vi "Strategy 5_Autotuning PID Offline.vi"() -> ()   [LabVIEW 2018]
doc: "This example demonstrates how to use the PID Design function to obtain PID parameters based on measured process."
uses:
  <vilib>/DAQmx/write.llb/DAQmx Write (Digital 1D Bool 1Chan 1Samp).vi
  <vilib>/addons/control/pid/autopid.llb/PID Autotuning Design (Ziegler-Nichols).vi
  <vilib>/addons/control/pid/autopid.llb/PID Autotuning Design (Cohen-Coon).vi
  <vilib>/addons/control/pid/autopid.llb/PID Autotuning Design (Chien-Hrones-Reswick).vi
  <vilib>/addons/control/pid/autopid.llb/PID Autotuning Design (Internal Model Control).vi
  <vilib>/DAQmx/create/channels.llb/DAQmx Create Channel (DO-Digital Output).vi
  <vilib>/addons/control/pid/pid.llb/PID Advanced (DBL).vi
  <vilib>/DAQmx/miscellaneous.llb/DAQmx Fill In Error Info.vi
  <vilib>/addons/control/pid/NI_PID_autopid.lvlib
  <vilib>/addons/control/pid/NI_PID_pid.lvlib
  <vilib>/ptbypt/NI_PtbyPt.lvlib
panel:
  out "PWM Output":bool
  out "Waveform Chart 2":dbl[][](graph)
  in  "MV:":dbl(slide)=20.39115328927357 scale=-100.0..100.0
  in  "Set\nPoint":dbl(slide) scale=0.0..30.0
  out "Waveform Chart":dbl[][](graph)
  in  "sample length":i32=100
  in  "Excitation":dbl=0.5 format="%.2f"
  in  "Type of controller":u16(ring)=2 items=["P", "PI", "PID"]
  in  "Control":T1(tab)
  in  "Ziegler-Nichols speed":u16(ring) items=["Fast", "Normal", "Slow"]
  in  "Tuning specifications":u16(ring) items=["Regulator - 0 %", "Regulator -  20%", "Servo - 0%", "Servo - 20%"]
  in  "Multiplicative factor":dbl(slide)=1.0 scale=0.01..100.0
  in  "Tab Control":T2(tab)
  in  "Instructions":string="Overview: This example demonstrates how to use the PID Autotuning Design to obtain PID parameters based on setpoint and process variable collected in another loop.\nInstructions:\n1. Run the VI and wait until the process variable (PV) reaches near setpoint (SP).\n2.  In the PID Autotuning Design section, select the type of algorithm, type of controller and excitation amplitude for the 'open loop step response'. Then, click Autotune to start the process. Select the Identified Plant Parameter tab and see the results from the identification.\n3.  When the tuned PID gains do not change anymore, the identification is done and you have the option to accept by clicking Accept gain, which will transfer the new gain to PID Gains.\n4. Click the Autotune button again to go back to the automatic control state. You can try different options and repeat this process.\n5. Click Stop to stop the VI.\n"
  out "Identified Plant Parameters":T3={"Plant Gain (K)"=1.7609511324977591, "Time Constant (T)"=1.9621978490901302, "Dead Time (L)"=0.22467425343567116}
  out "Control Output":dbl[](graph)
  out "Measurement":dbl[](graph)
  out "Stimulus operating point":dbl=20.314221540357543
  out "Response operating point":dbl=51.08345461694337
  in  "Automatic":bool=TRUE
  in  "Reinitialize":bool
  out "MV":dbl(graph)=20.39115328927357
  in  "Accept gain":bool
  out "Tuned PID gains":T4={"proportional gain (Kc)"=1.9838195929127882, "integral time (Ti, min)"=0.01995856284686879, "derivative time (Td, min)"=0.0} {"derivative time (Td, min)" format="%#.6g"; "integral time (Ti, min)" format="%#.6g"; "proportional gain (Kc)" format="%#.6g"}
  in  "Autotune":bool
  in  "PID Gains":T4={"proportional gain (Kc)"=2.5, "integral time (Ti, min)"=0.02, "derivative time (Td, min)"=0.0} {"derivative time (Td, min)" format="%#.6g"; "integral time (Ti, min)" format="%#.6g"; "proportional gain (Kc)" format="%#.6g"}
  in  "Sampling Time dt (s)":dbl=0.05 min=0.001 step=0.01 format="%#.3p"
  in  "Stop":bool
  # "Proportional-Integral-Derivative (PID) Controller"
  # "PID Autotuning Design"
  # "No additional parameters"
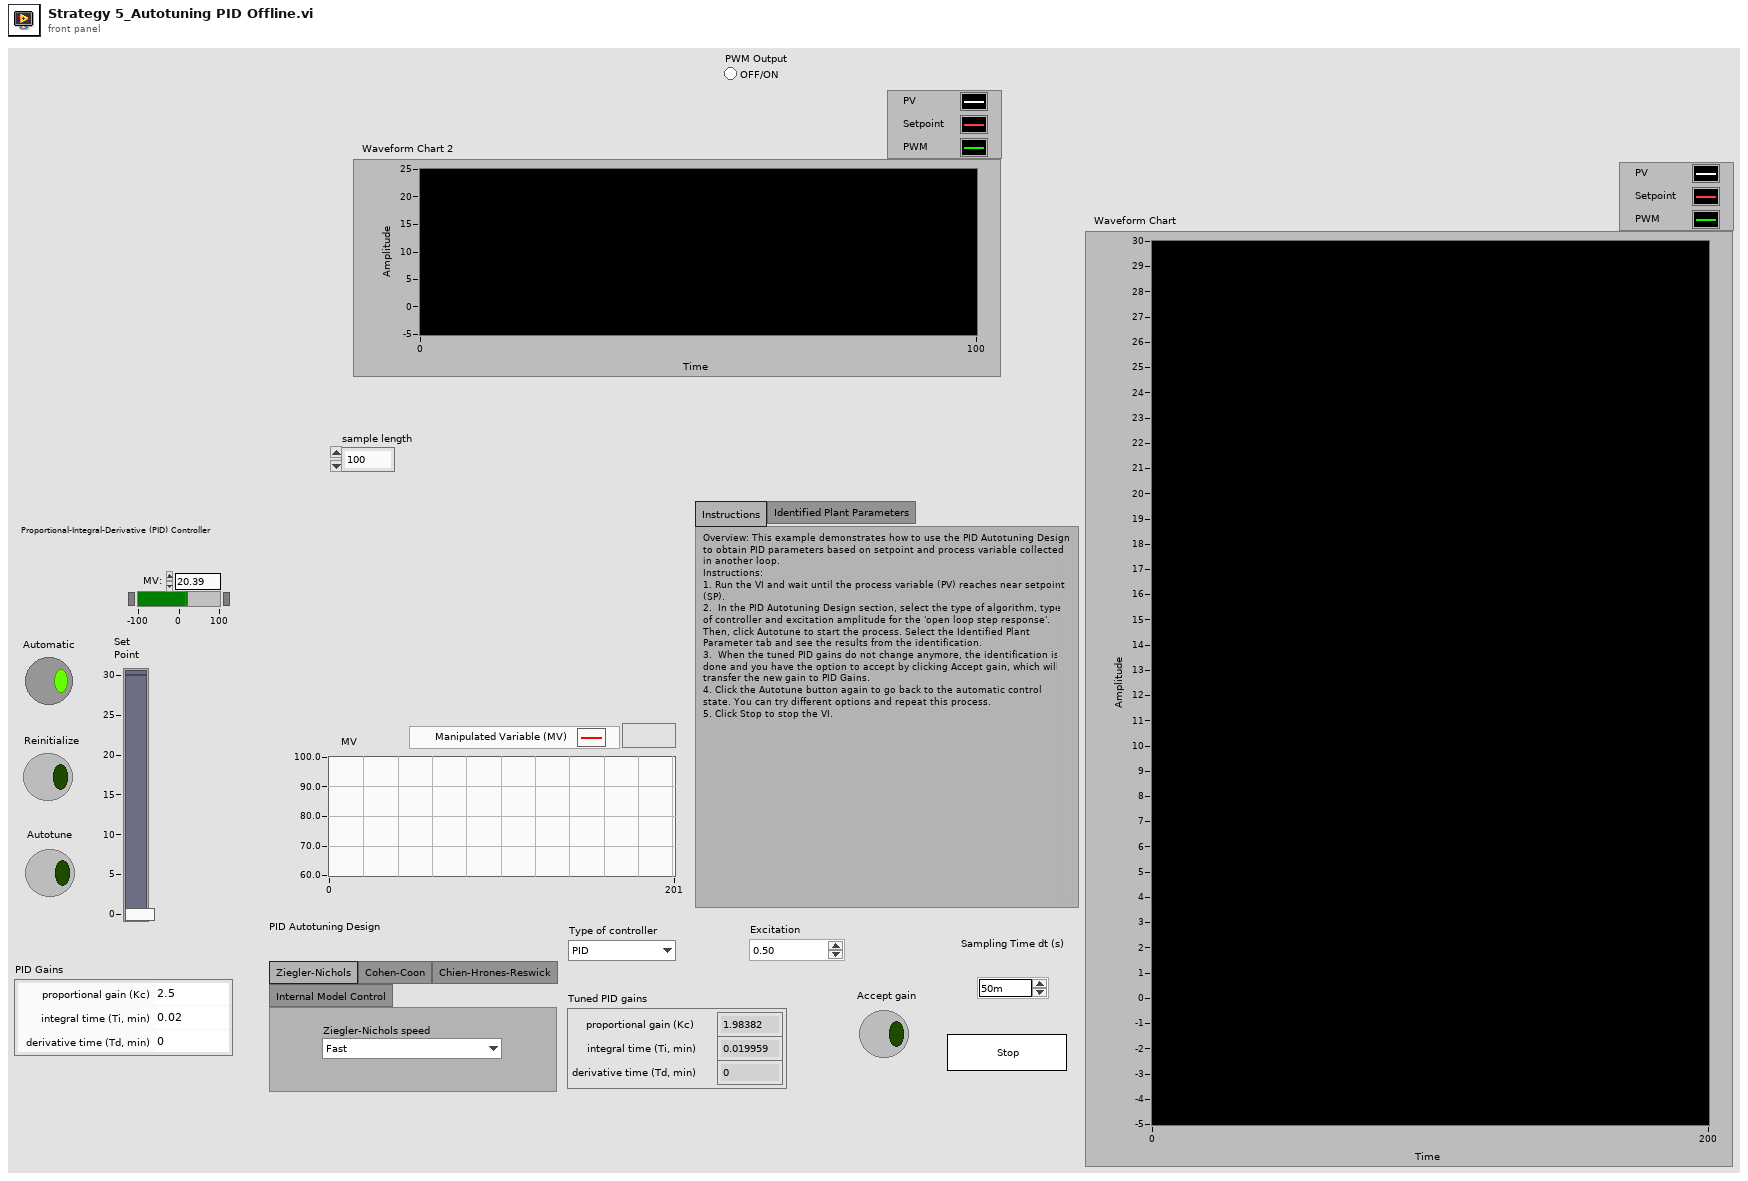
[diagram p1: front panel]
types:
  T1 = enum32{"Ziegler-Nichols", "Cohen-Coon", "Chien-Hrones-Reswick", "Internal Model Control"}
  T2 = enum32{"Instructions", "Identified Plant Parameters"}
  T3 = cluster{"Plant Gain (K)":dbl, "Time Constant (T)":dbl, "Dead Time (L)":dbl}
  T4 = cluster{"proportional gain (Kc)":dbl, "integral time (Ti, min)":dbl, "derivative time (Td, min)":dbl}
  T5 = cluster{"static gain":dbl, "lag (s)":dbl, "deadtime (s)":dbl, "load":dbl, "deadband":dbl, "sensor noise":dbl, "initial PV":dbl, "plant noise":dbl}
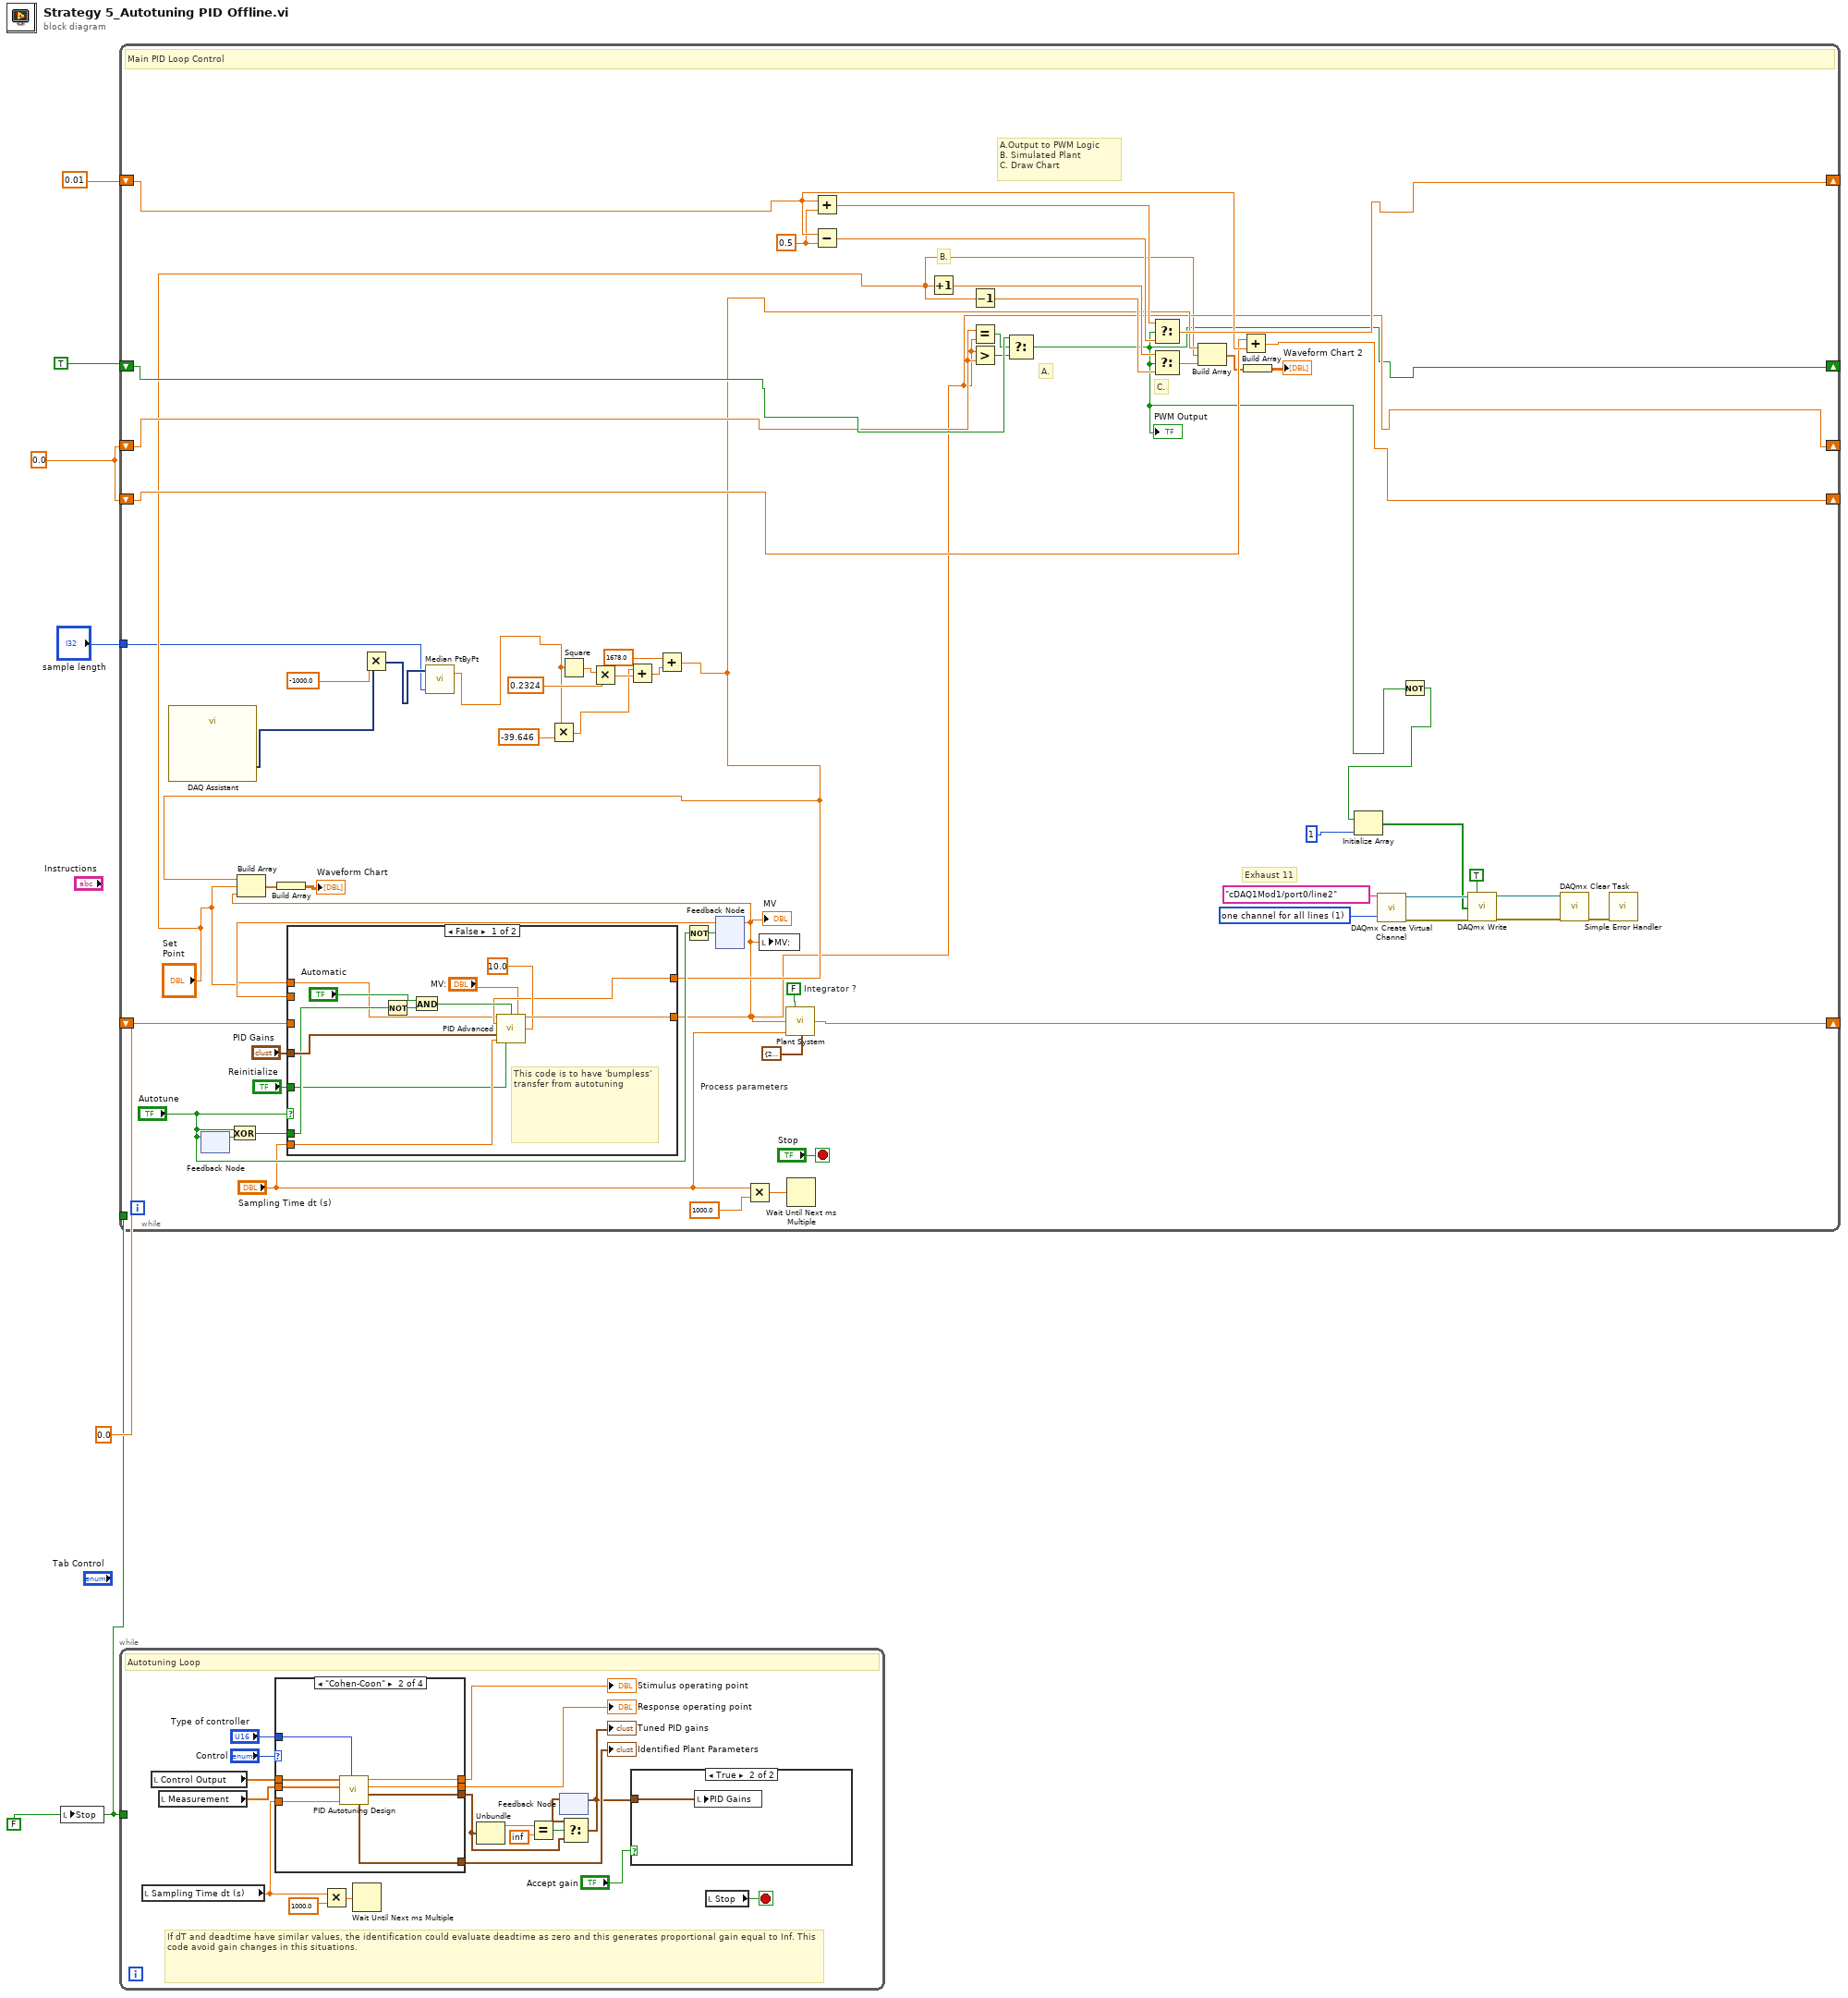
[diagram p0: block diagram]
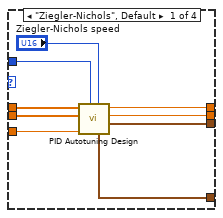
[diagram p2: hidden frame]
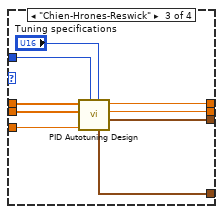
[diagram p3: hidden frame]
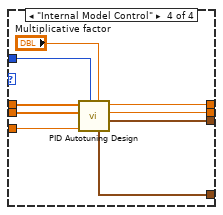
[diagram p4: hidden frame]
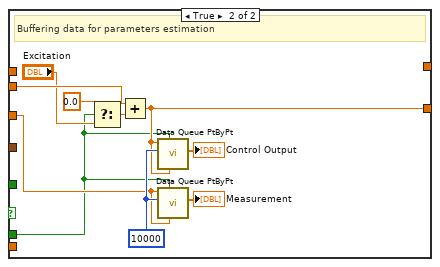
[diagram p6: hidden frame]
diagram:
  w2 = 0.0 ("output")
  w5 = FALSE ("Stop")
  n1 = local write "Stop"(w5) -> ()
  n2 = while {
    shift-left: 0.0 ("Plant Output") -> [w61]
    shift-right: [w56] -> _
    tunnel: w5 -> [_]
    shift-right: [w38] -> _
    shift-left: 0.01 -> [w36]
    shift-right: [w8] -> _
    shift-left: TRUE -> [w35]
    shift-right: [w11] -> _
    shift-left: w2 -> [w34]
    shift-right: [w37] -> _
    shift-left: w2 -> [w33]
    tunnel: "sample length" -> [w9]
    stop <- "Stop" stop-if-true
    w16 = 1 items=["one channel for each line", "one channel for all lines"] ("line grouping")
    w24 = 0.5 ("x")
    w55 = T5 {"static gain"=2.5, "lag (s)"=2.5, "deadtime (s)"=0.01, "load"=0.0, "deadband"=0.0, "sensor noise"=0.0, "initial PV"=30.0, "plant noise"=0.0}  # Process parameters
    w57 = FALSE  # Integrator ?
    # "Exhaust 11"
    # "B."
    # "C."
    # "A."
    # "A.Output to PWM Logic \nB. Simulated Plant\nC. Draw Chart"
    # "Main PID Loop Control"
    n3 = call "DAQ Assistant"() -> ("data"=w51:dynamicdata)  [unwired: 17 in, 2 out]
    n4 = feedback #1() -> (w63:bool)  [unwired: 1 in]
    n5 = feedback-in #1("Autotune") -> ()
    n6 = Exclusive Or(1:w63, 2:"Autotune") -> (0:w62:bool)
    n7 = Multiply(x=w51, y=-1000.0) -> (x*y=w42:dynamicdata)
    n8 = call <vilib>:"Median PtByPt.vi"("sample length"=w9, "x"=w42) -> ("median"=w41:dbl)  [unwired: 2 in, 1 out]
    n9 = Multiply(x=w41, y=-39.646) -> (x*y=w45:dbl)
    n10 = Square(x=w41) -> (x^2=w49:dbl)
    n11 = Multiply(x=w49, y=0.2324) -> (x*y=w46:dbl)
    n12 = Add(x=w45, y=w46) -> (x+y=w44:dbl)
    n13 = Add(x=1678.0, y=w44) -> (x+y=w12:dbl)
    n14 = Not(x="Autotune") -> (.not. x?=w58:bool)
    n15 = feedback #2() -> (w60:dbl)  [unwired: 1 in]
    n16 = case shown="False" "Autotune" {
      tunnel: "Sampling Time dt (s)" -> [w78 _]
      tunnel: [w76 w81] -> w11
      tunnel: w61 -> [_ w80]
      tunnel: "PID Gains" -> [w77 _]
      tunnel: "Reinitialize" -> [w73 _]
      tunnel: w62 -> [w75 w79]
      tunnel: w60 -> [_ w85]
      tunnel: w12 -> [w69 _]
      tunnel: "Set\nPoint" -> [w68 _]
      frame False {
        # "This code is to have 'bumpless' transfer from autotuning"
        n17 = Not(x=w75) -> (.not. x?=w72:bool)
        n18 = And(x="Automatic", y=w72) -> (x .and. y?=w74:bool)
        n19 = call-poly <vilib>:"PID Advanced.vi"("setpoint"=w68, "auto? (T)"=w74, "manual control"="MV:", "process variable"=w69, "alpha"=10.0, "PID gains"=w77, "dt (s)"=w78, "reinitialize? (F)"=w73) -> ("output"=w76:dbl)  [unwired: 6 in, 1 out]
      }
      frame True {
        w88 = 10000 ("sample length")
        # "Buffering data for parameters estimation"
        n20 = Select(t=0.0, s=w79, f="Excitation") -> (s? t:f=w86:dbl)
        n21 = Add(x=w85, y=w86) -> (x+y=w81:dbl)
        n22 = call <vilib>:"Data Queue PtByPt.vi"("initial queue element"=w81, "initialize"=w79, "sample length"=w88, "input data point"=w81) -> ("Current Queue"=→"Control Output":dbl[])  [unwired: 3 in, 4 out]
        n23 = call <vilib>:"Data Queue PtByPt.vi"("initial queue element"=w80, "initialize"=w79, "sample length"=w88, "input data point"=w80) -> ("Current Queue"=→"Measurement":dbl[])  [unwired: 3 in, 4 out]
      }
    }
    "MV" <- w11
    n24 = Build Array(w12, "Set\nPoint", w11) -> (w39:dbl[])
    n25 = Build Array(w39) -> (→"Waveform Chart":dbl[][])
    n26 = feedback-in #2(w11, w58) -> ()
    n27 = Multiply(x="Sampling Time dt (s)", y=1000.0) -> (x*y=w53:dbl)
    n28 = local write "MV:"(w11) -> ()
    n29 = call "Plant System.vi"("Integrator ?"=w57, "Plant Input"=w11, "dt (s)"="Sampling Time dt (s)", "process parameters"=w55) -> ("Plant Output"=w56:dbl)  [unwired: 11 in]
    n30 = Wait Until Next ms Multiple(millisecond multiple=w53) -> ()  [unwired: 1 out]
    n31 = Add(x=w36, y=w24) -> (x+y=w25:dbl)
    n32 = Subtract(x=w36, y=w24) -> (x-y=w23:dbl)
    n33 = Increment(x="Set\nPoint") -> (x+1=w29:dbl)
    n34 = Decrement(x="Set\nPoint") -> (x-1=w28:dbl)
    n35 = Equal?(x=w34, y=w11) -> (x = y?=w31:bool)
    n36 = Greater?(x=w11, y=w34) -> (0:w30:bool)
    n37 = Select(t=w35, s=w31, f=w30) -> (s? t:f=w8:bool)
    "PWM Output" <- w8
    n38 = Select(t=w25, s=w8, f=w23) -> (s? t:f=w38:dbl)
    n39 = Select(t=w29, s=w8, f=w28) -> (s? t:f=w27:dbl)
    n40 = Build Array(w12, "Set\nPoint", w27) -> (w26:dbl[])
    n41 = Add(x=w33, y=w36) -> (x+y=w37:dbl)
    n42 = Build Array(w26) -> (→"Waveform Chart 2":dbl[][])
    n43 = call-poly <vilib>:"DAQmx Create Virtual Channel.vi"("lines"=tag "cDAQ1Mod1/port0/line2", "line grouping"=w16) -> ("task out"=w18:refnum<k21>, "error out"=w17:errorcluster)  [unwired: 12 in]
    n44 = Not(x=w8) -> (.not. x?=w7:bool)
    n45 = Initialize Array(w7, 1 ("dimension size")) -> (w13:bool[])
    n46 = call-poly <vilib>:"DAQmx Write.vi"("task/channels in"=w18, "auto start"=TRUE, "data"=w13, "error in"=w17) -> ("task out"=w20:refnum<k21>, "error out"=w21:errorcluster)  [unwired: 9 in, 1 out]
    n47 = call <vilib>:"DAQmx Clear Task.vi"("task in"=w20, "error in"=w21) -> ("error out"=w15:errorcluster)  [unwired: 13 in]
    n48 = call <vilib>:"Simple Error Handler.vi"("error in (no error)"=w15) -> ()  [unwired: 4 in, 5 out]
  }
  n49 = while {
    tunnel: w5 -> [_]
    stop <- w101 stop-if-true
    # "If dT and deadtime have similar values, the identification could evaluate deadtime as zero and this generates proportional gain equal to Inf. This code avoid gain changes in this situations."
    # "Autotuning Loop"
    n50 = local read "Sampling Time dt (s)"() -> (w102:dbl)
    n51 = local read "Control Output"() -> (w106:dbl[])
    n52 = local read "Measurement"() -> (w105:dbl[])
    n53 = case shown="\"Cohen-Coon\"" "Control" {
      tunnel: w106 -> [w115 w123 w132 w141]
      tunnel: w105 -> [w114 w122 w131 w140]
      tunnel: [w113 w121 w130 w139] -> w104
      tunnel: [w112 w120 w129 w138] -> w103
      tunnel: w102 -> [w111 w119 w128 w137]
      tunnel: [w110 w118 w127 w136] -> w99
      tunnel: [w109 w117 w126 w135] -> w90
      tunnel: "Type of controller" -> [w108 w116 w125 w134]
      frame "Ziegler-Nichols", Default {
        n54 = call-poly <vilib>:"PID Autotuning Design.vi"("Ziegler-Nichols Speed"="Ziegler-Nichols speed", "Type of Controller"=w108, "dt (s)"=w111, "Response signal"=w114, "Stimulus signal"=w115) -> ("PID gains"=w109:T4, "response operating point"=w112:dbl, "stimulus operating point"=w113:dbl, "Plant Parameters"=w110:T3)  [unwired: 3 in]
      }
      frame "Cohen-Coon" {
        n55 = call-poly <vilib>:"PID Autotuning Design.vi"("Type of Controller"=w116, "dt (s)"=w119, "Response signal"=w122, "Stimulus signal"=w123) -> ("PID gains"=w117:T4, "response offset"=w120:dbl, "stimulus offset"=w121:dbl, "Plant Parameters"=w118:T3)  [unwired: 4 in]
      }
      frame "Chien-Hrones-Reswick" {
        n56 = call-poly <vilib>:"PID Autotuning Design.vi"("Tuning specifications"="Tuning specifications", "Type of Controller"=w125, "dt (s)"=w128, "Response signal"=w131, "Stimulus signal"=w132) -> ("PID gains"=w126:T4, "response offset"=w129:dbl, "stimulus offset"=w130:dbl, "Plant Parameters"=w127:T3)  [unwired: 3 in]
      }
      frame "Internal Model Control" {
        n57 = call-poly <vilib>:"PID Autotuning Design.vi"("Desired Time Constant (tau_c)"="Multiplicative factor", "Type of Controller"=w134, "dt (s)"=w137, "Response signal"=w140, "Stimulus signal"=w141) -> ("PID gains"=w135:T4, "response offset"=w138:dbl, "stimulus offset"=w139:dbl, "Plant Parameters"=w136:T3)  [unwired: 3 in]
      }
    }
    "Stimulus operating point" <- w104
    "Response operating point" <- w103
    "Identified Plant Parameters" <- w99
    n58 = Multiply(x=w102, y=1000.0) -> (x*y=w98:dbl)
    n59 = Wait Until Next ms Multiple(millisecond multiple=w98) -> ()  [unwired: 1 out]
    n60 = Unbundle(w90) -> ("proportional gain (Kc)"=w93:dbl)  [unwired: 2 out]
    n61 = Equal?(x=w93, y=inf) -> (x = y?=w92:bool)
    n62 = feedback #3() -> (w91:T4)  [unwired: 1 in]
    n63 = Select(t=w91, s=w92, f=w90) -> (s? t:f=w89:T4)
    "Tuned PID gains" <- w89
    n64 = feedback-in #3(w89) -> ()
    n65 = case shown="True" "Accept gain" {
      tunnel: w89 -> [_ w142]
      frame False {
      }
      frame True {
        n66 = local write "PID Gains"(w142) -> ()
      }
    }
    n67 = local read "Stop"() -> (w101:bool)
  }
